vi "Measurement UI.vi"() -> ()   [LabVIEW 2025, in "Workflow DO UI.lvlib"]
uses:
  Workflow DO UI.lvlib
panel:
  out "CAN Error":bool
  out "Message Buffer":string[][](table)
  in  "TYPE":u32(ring) items=["CAN Data"=0, "CAN Remote"=1, "CAN Bus Error"=2, "CAN 2.0 Data"=8, "CAN FD Data"=16, "CAN FD+BRS Data"=24, "J1939 Data"=192, "Delay"=224, "Log Trigger"=225, "Start Trigger"=226]
  in  "CAN Interface Name":string
  in  "Termination CAN":bool
  out "Timeout":bool
  out "Count":u32
  out "Trace":string[][](table)
  out "Digital Input":u32[](graph)
  in  "IO Mode":enum32{"CAN", "CAN FD", "CAN FD + BRS"}(ring)
  in  "FD ISO Mode":enum32{"ISO", "Legacy ISO", "Non-ISO"}(ring)=enum."Non-ISO"
  in  "Baudrate":u32=125000 format="%x"
  in  "FD Baudrate":u32 format="%x"
  in  "INTERFACE NAME CAN":refnum<k21>="CAN1"
  in  "PAYLOAD":u32[](array[numeric])=[0, 1, 2, 3, 4, 5, 6, 7] format="%x"
  in  "IDENTIFIER":u32=1034 format="%x"
  in  "Timeout (s)":u32=30
  in  "Pulses":u32=20
  in  "Counter Interface":string
  in  "Input Terminal Name":string
  in  "Active Edge":i32(ring)=10171 items=["Rising"=10280, "Falling"=10171]
  in  "Input Terminal":tag="/PXI1Slot6/PFI0"
  in  "Counter":tag="PXI1Slot6/ctr0"
  # "CAN Settings"
  # "Digital Channel Settings"
  # "Number of Expected Pulses"
  # "CAN Trace"
  # "Results"
  # "Counter"
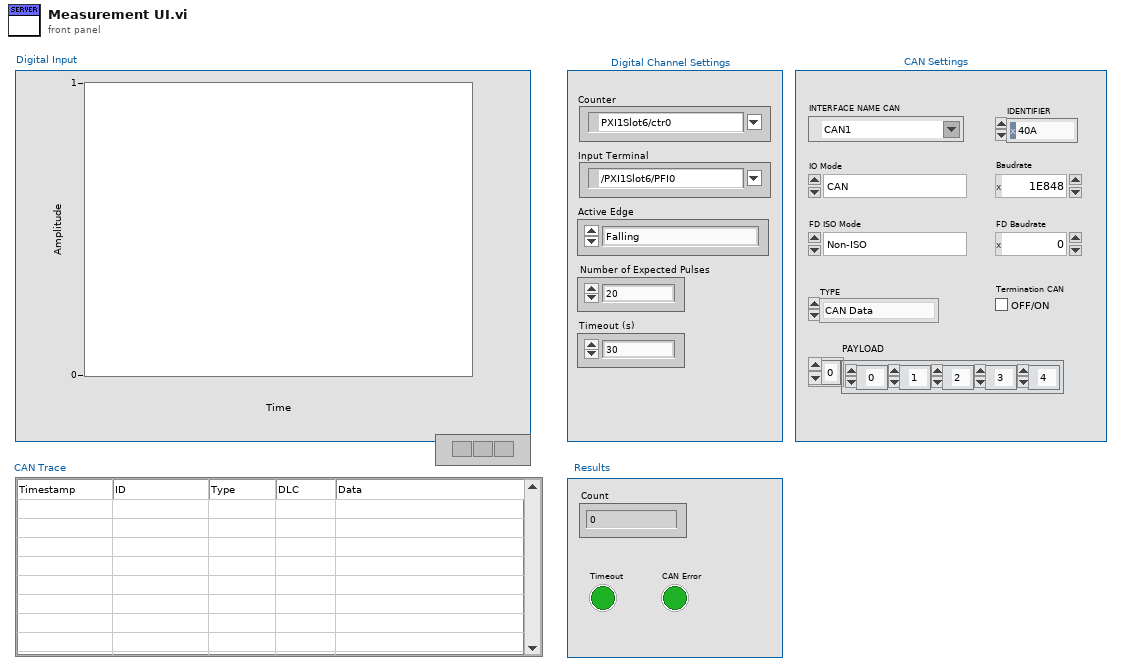
[diagram p1: front panel]
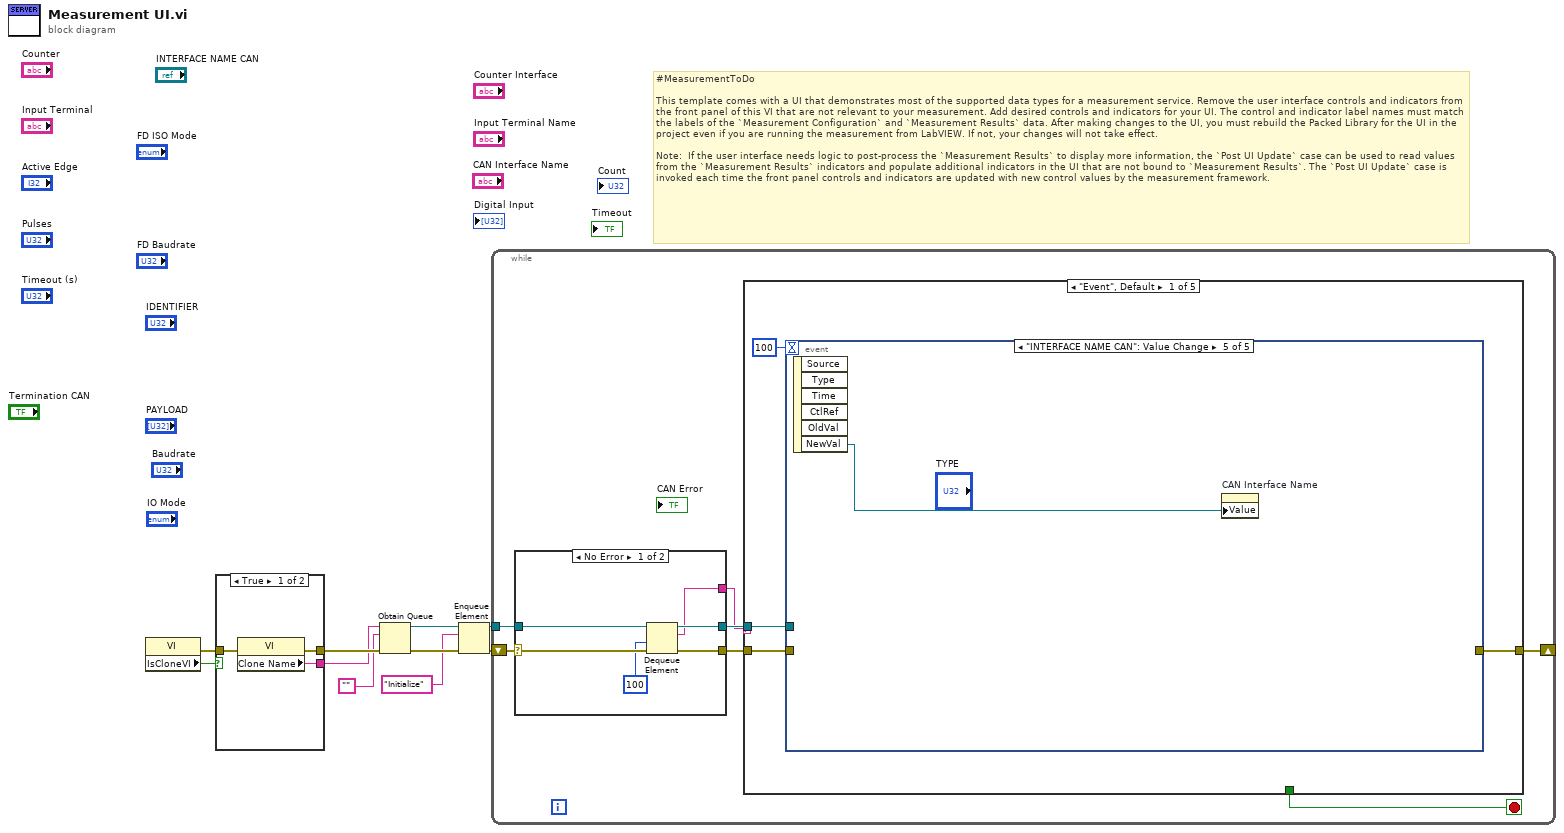
[diagram p0: block diagram]
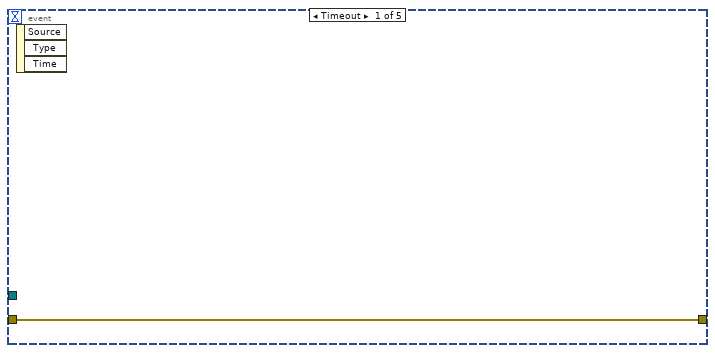
[diagram p2: hidden frame]
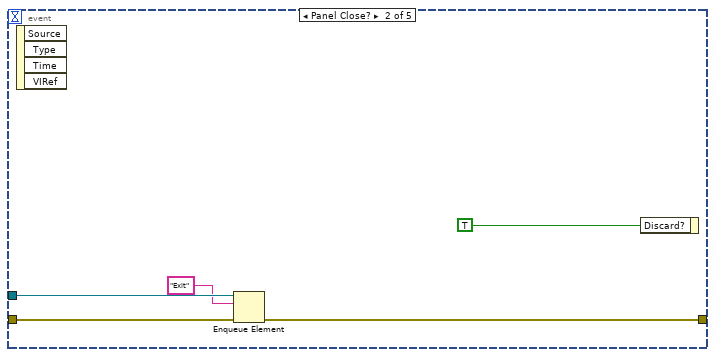
[diagram p3: hidden frame]
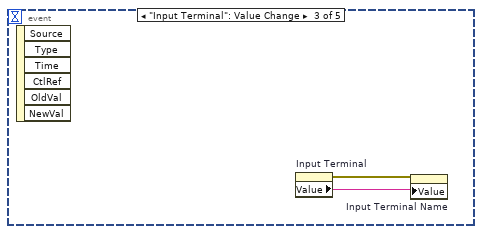
[diagram p4: hidden frame]
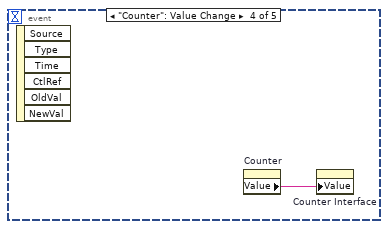
[diagram p5: hidden frame]
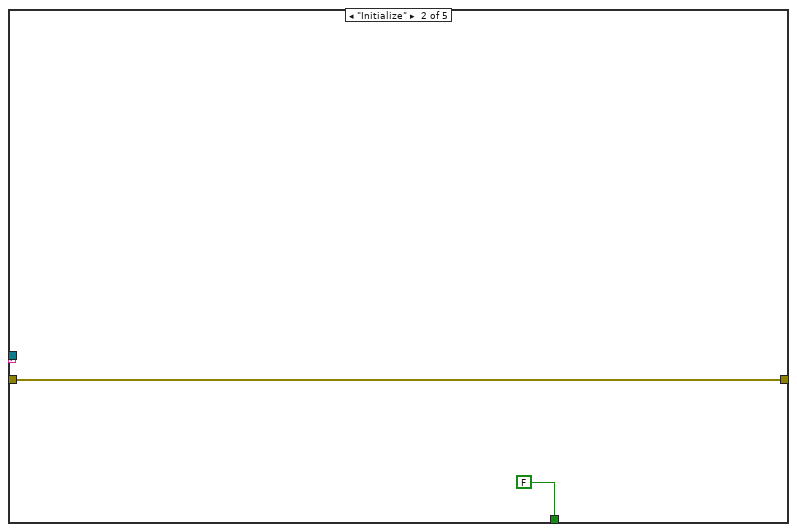
[diagram p6: hidden frame]
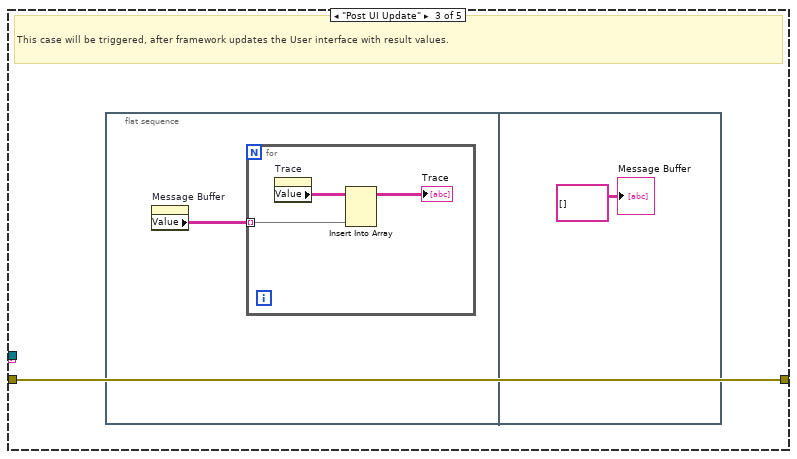
[diagram p7: hidden frame]
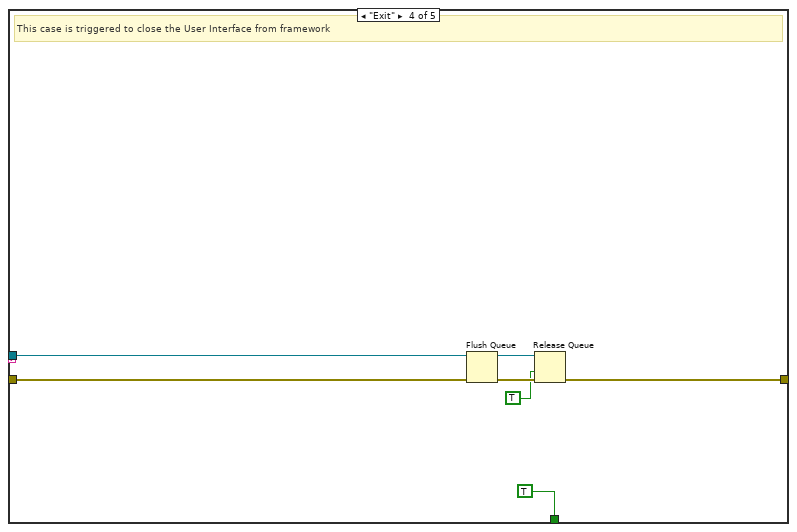
[diagram p8: hidden frame]
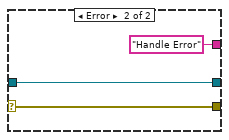
[diagram p10: hidden frame]
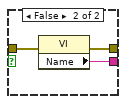
[diagram p11: hidden frame]
diagram:
  # "#MeasurementToDo  \n\nThis template comes with a UI that demonstrates most of the supported data types for a measurement service. Remove the user interface controls and indicators from the front panel of this VI that are not relevant to your measurement. Add desired controls and indicators for your UI. The control and indicator label names must match the labels of the `Measurement Configuration` and `Measurement Results` data. After making changes to the UI, you must rebuild the Packed Library for the UI in the project even if you are running the measurement from LabVIEW. If not, your changes will not take effect.\n\nNote:  If the user interface needs logic to post-process the `Measurement Results` to display more information, the `Post UI Update` case can be used to read values from the `Measurement Results` indicators and populate additional indicators in the UI that are not bound to `Measurement Results`. The `Post UI Update` case is invoked each time the front panel controls and indicators are updated with new control values by the measurement framework."
  n1 = property class="VI"() -> (error out=w1:errorcluster, "IsCloneVI"=w2:bool)  [unwired: 2 in, 1 out]
  n2 = case shown="True" w2 {
    tunnel: [w13 w16] -> w10
    tunnel: [w12 w15] -> w9
    tunnel: w1 -> [w11 w14]
    frame True {
      n3 = property class="VI"(error in=w11) -> (error out=w13:errorcluster, "Clone Name"=w12:string)  [unwired: 1 in, 1 out]
    }
    frame False {
      n4 = property class="VI"(error in=w14) -> (error out=w16:errorcluster, "Name"=w15:string)  [unwired: 1 in, 1 out]
    }
  }
  n5 = Obtain Queue(name (unnamed)=w9, element data type="", error in (no error)=w10) -> (queue out=w6:refnum<queue>, error out=w8:errorcluster)  [unwired: 2 in, 1 out]
  n6 = Enqueue Element(queue=w6, element="Initialize", error in (no error)=w8) -> (queue out=w5:refnum<queue>, error out=w7:errorcluster)  [unwired: 1 in, 1 out]
  n7 = while {
    shift-right: [w18] -> _
    shift-left: w7 -> [w23]
    tunnel: w5 -> [w21]
    stop <- w17 stop-if-true
    n8 = case shown="No Error" w23 {
      selector: w23 -> [w59 w62]
      tunnel: [w58 w62] -> w22
      tunnel: w21 -> [w57 w61]
      tunnel: [w56 w61] -> w20
      tunnel: [w55 "Handle Error"] -> w19
      frame No Error {
        n9 = Dequeue Element(queue=w57, timeout in ms (-1)=100, error in (no error)=w59) -> (queue out=w56:refnum<queue>, element=w55:string, error out=w58:errorcluster)  [unwired: 1 out]
      }
      frame Error {
      }
    }
    n10 = case shown="\"Event\", Default" w19 {
      tunnel: w22 -> [w26 w39 w40 w52 w53]
      tunnel: w20 -> [w24 _ _ w50 _]
      tunnel: [w27 w39 w40 w47 w53] -> w18
      tunnel: [_ FALSE _ TRUE _] -> w17
      frame "Event", Default {
        n11 = event shown="[4] \"INTERFACE NAME CAN\": Value Change" {
          selector: _ -> [_ _ _ _ _]
          dyn-events: _ -> [_ _ _ _ _]
          timeout: 100 -> [_ _ _ _ _]
          tunnel: [w28 w31 _ _ _] -> w27
          tunnel: w26 -> [w28 w32 _ _ _]
          tunnel: w24 -> [_ w30 _ _ _]
          event Timeout {
            n12 = event-data() -> ()  [unwired: 1 in, 3 out]
          }
          event Panel Close? {
            n13 = event-data() -> ()  [unwired: 1 in, 4 out]
            n14 = Enqueue Element(queue=w30, element="Exit", error in (no error)=w32) -> (error out=w31:errorcluster)  [unwired: 1 in, 2 out]
            n15 = event-data("Discard?"=TRUE) -> ()  [unwired: 1 in, 1 out]
          }
          event "Input Terminal": Value Change {
            n16 = event-data() -> ()  [unwired: 1 in, 6 out]
            n17 = property on="Input Terminal" class="DAQmxName"() -> (error out=w34:errorcluster, "Value"=w35:string)  [unwired: 2 in, 1 out]
            n18 = property on="Input Terminal Name" class="Str"(error in=w34, "Value"=w35) -> ()  [unwired: 1 in, 2 out]
          }
          event "Counter": Value Change {
            n19 = event-data() -> ()  [unwired: 1 in, 6 out]
            n20 = property on="Counter" class="DAQmxName"() -> ("Value"=w36:string)  [unwired: 2 in, 2 out]
            n21 = property on="Counter Interface" class="Str"("Value"=w36) -> ()  [unwired: 2 in, 2 out]
          }
          event "INTERFACE NAME CAN": Value Change {
            n22 = event-data() -> ("NewVal"=w37:refnum<k21>)  [unwired: 1 in, 5 out]
            n23 = property on="CAN Interface Name" class="Str"("Value"=w37) -> ()  [unwired: 2 in, 2 out]
          }
        }
      }
      frame "Initialize" {
      }
      frame "Post UI Update" {
        # "This case will be triggered, after framework updates the User interface with result values."
        n24 = flat-sequence {
          frame #0 {
            n25 = property on="Message Buffer" class="Tbl (strict)"() -> ("Value"=w41:string[][])  [unwired: 2 in, 2 out]
            n26 = for {
              tunnel: w41 -> [w43] mode=indexing
              n27 = property on="Trace" class="Tbl (strict)"() -> ("Value"=w44:string[][])  [unwired: 2 in, 2 out]
              n28 = Insert Into Array(array=w44, new element=w43) -> (→"Trace":string[][])  [unwired: 2 in]
            }
          }
          frame #1 {
            "Message Buffer" <- string[][] [] ("Message Buffer")
          }
        }
      }
      frame "Exit" {
        # "This case is triggered to close the User Interface from framework"
        n29 = Flush Queue(queue=w50, error in (no error)=w52) -> (queue out=w49:refnum<queue>, error out=w48:errorcluster)  [unwired: 1 out]
        n30 = Release Queue(queue=w49, force destroy? (F)=TRUE, error in (no error)=w48) -> (error out=w47:errorcluster)  [unwired: 2 out]
      }
      frame "Handle Error" {
      }
    }
  }
